vi "ShoreDefinition3.vi"(0 "Image In":T1, 7 "error in":errorcluster) -> (20 "Image Out":T1, 27 "error out":errorcluster)   [LabVIEW 2014]
uses:
  <vilib>/vision/Image Controls.llb/IMAQ Image.ctl
  <vilib>/vision/NI_Vision_Development_Module.lvlib
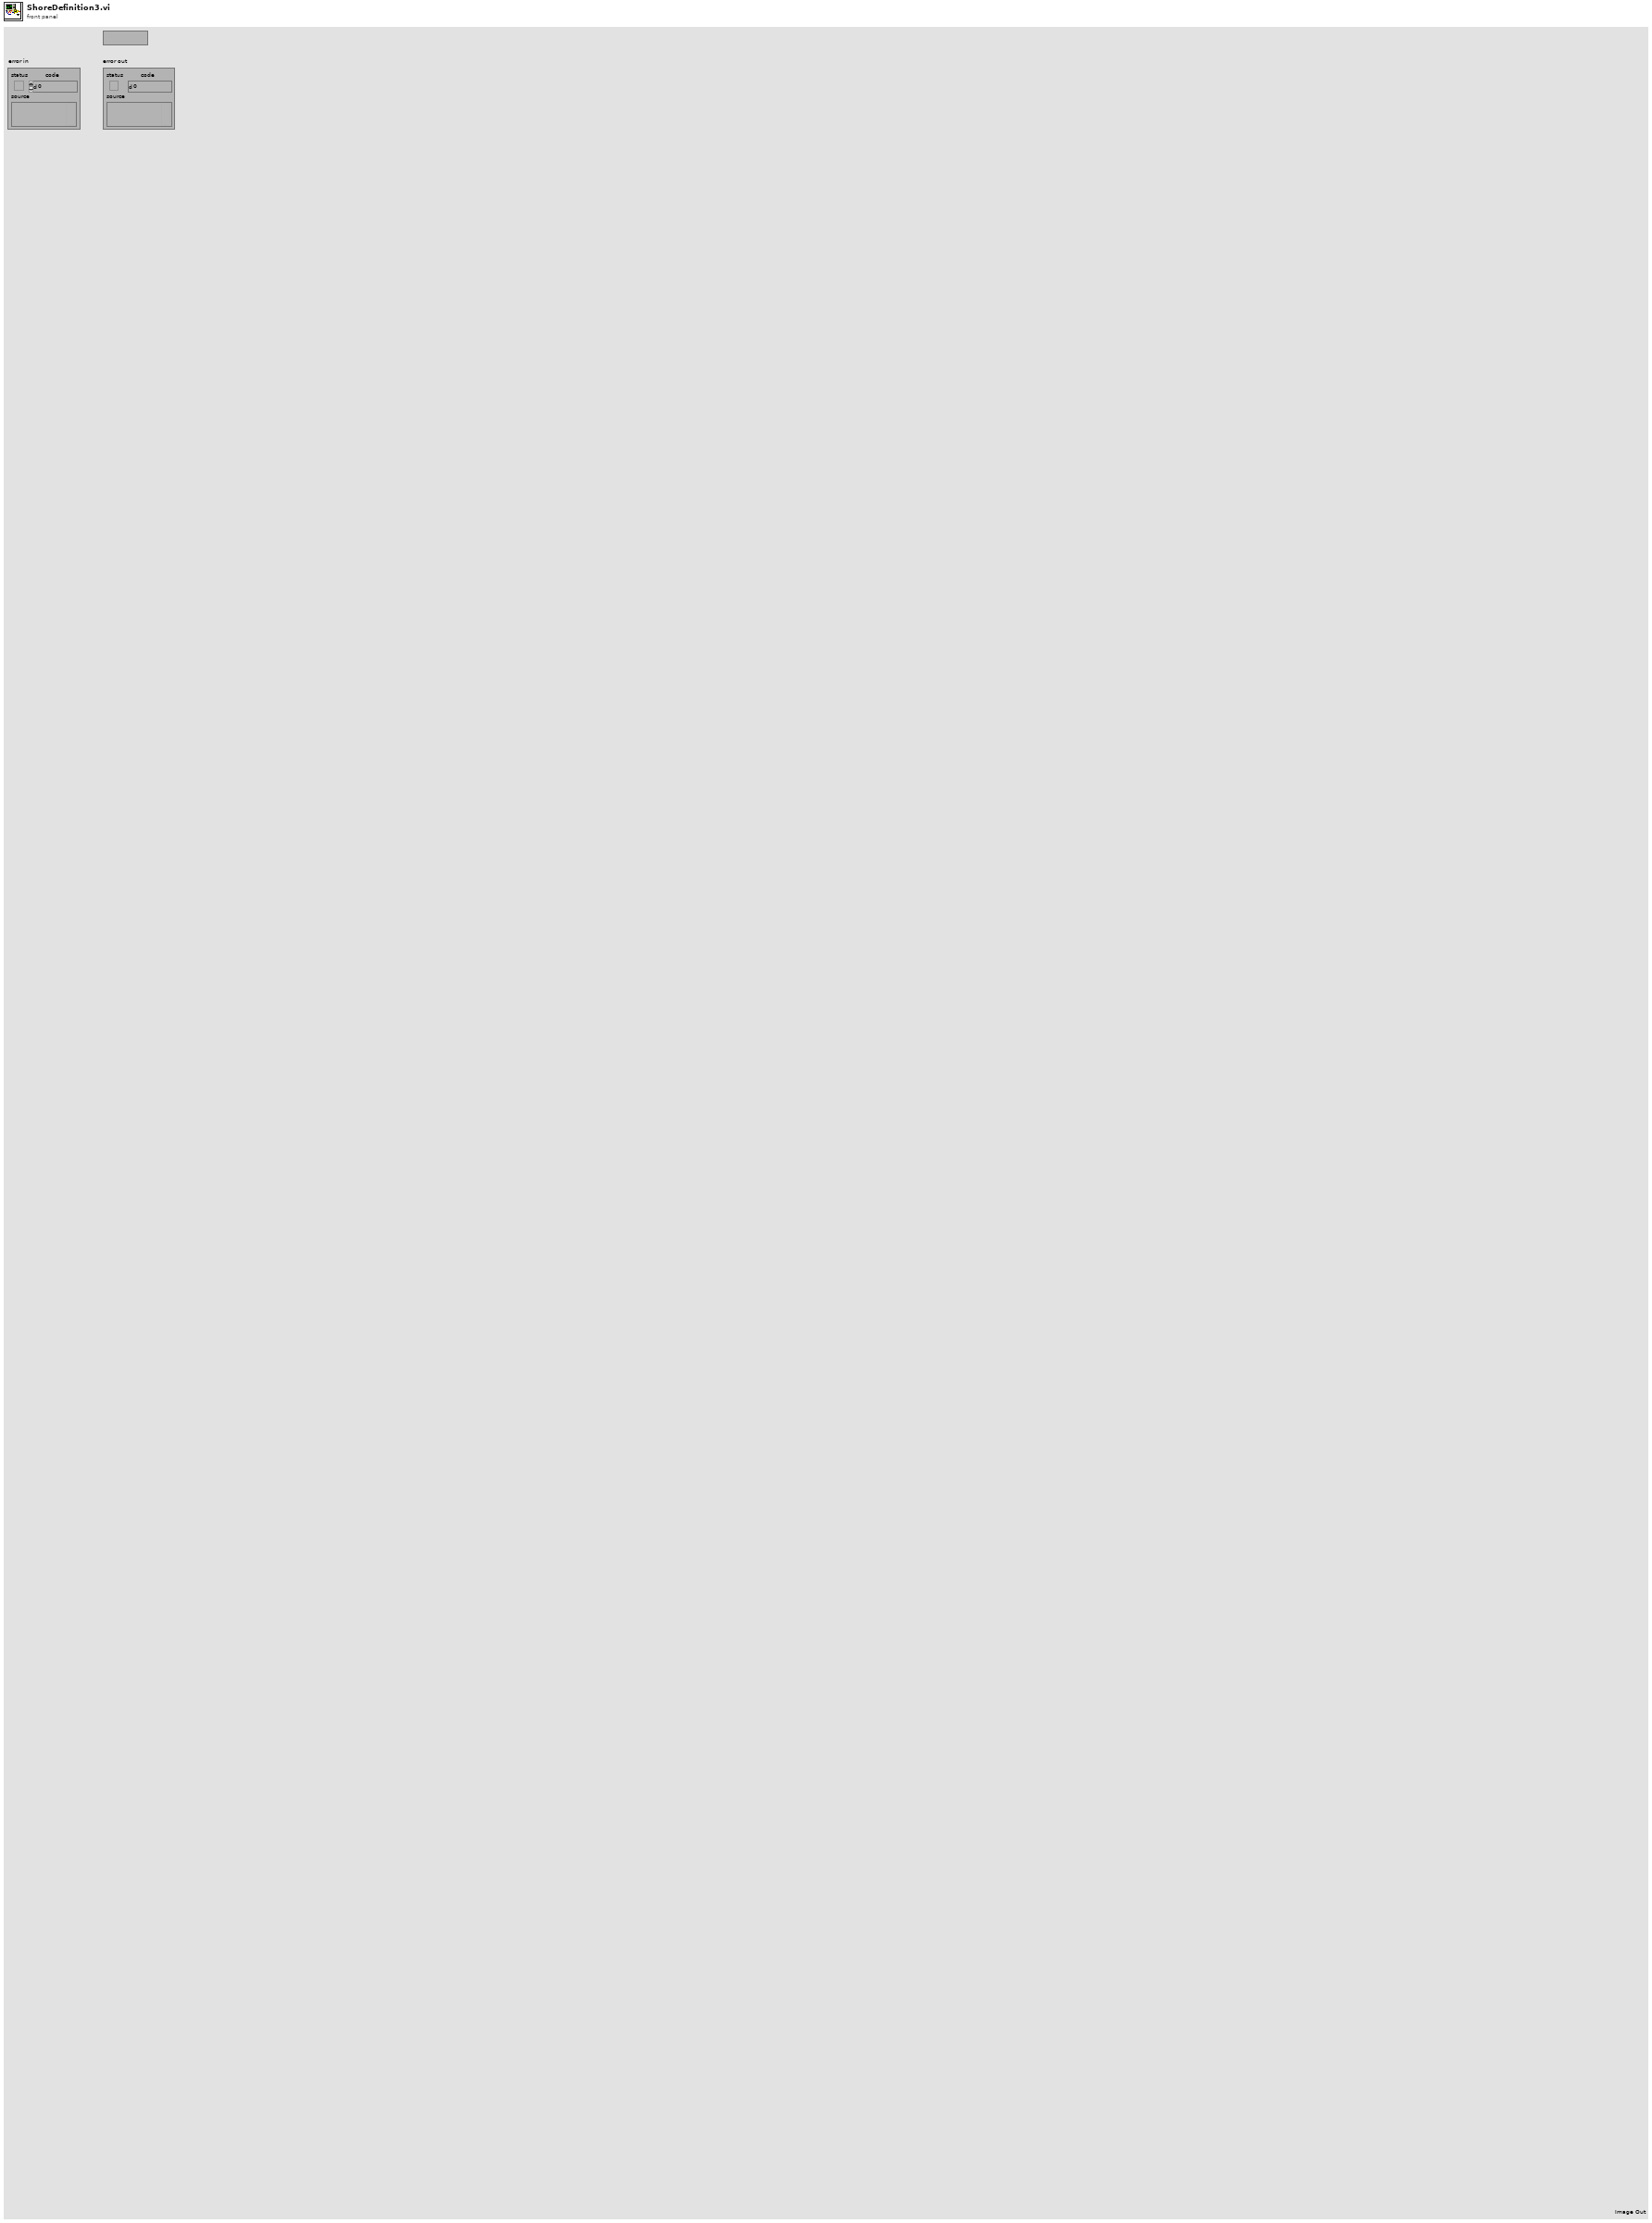
[diagram p1: front panel]
types:
  T1 = typedef "IMAQ Image.ctl" = refnum<image>
  T2 = enum32{"AutoM", "Close", "Dilate", "Erode", "Gradient", "Gradient out", "Gradient in", "Hit miss", "Open", "PClose", "POpen", "Thick", "Thin"}
  T3 = typedef "Image Type" = u32
  T4 = cluster{"Brightness":sgl, "Contrast":sgl, "Gamma":sgl}
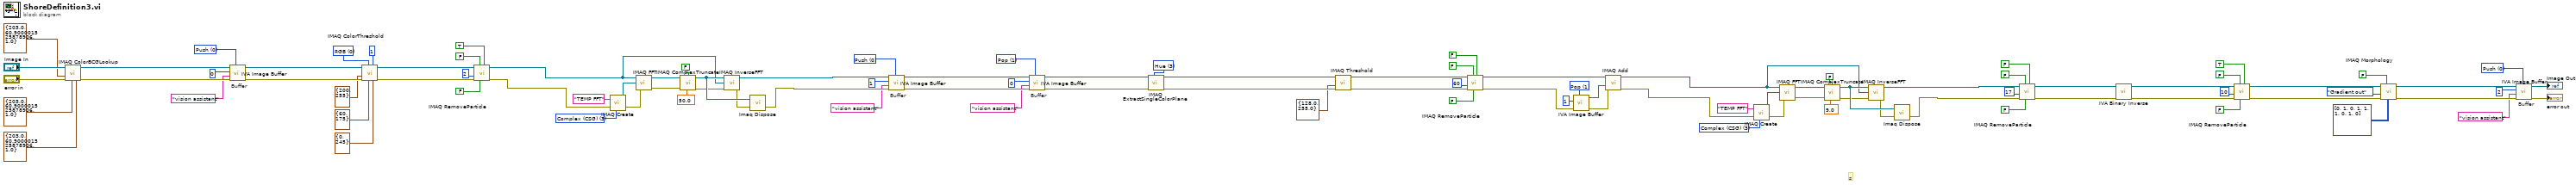
[diagram p0: block diagram]
diagram:
  w4 = u16 0 items=["Push", "Pop", "Reset"] ("Function")
  w26 = T3 3 items=["Grayscale (U8)", "Grayscale (I16)", "Grayscale (SGL)", "Complex (CSG)", "RGB (U32)", "HSL (U32)", "RGB (U64)", "Grayscale (U16)"] ("Image Type")
  w44 = u16 1 items=["Push", "Pop", "Reset"] ("Function")
  w56 = 3 items=["Red", "Green", "Blue", "Hue", "Saturation", "Luminance", "Value", "Intensity"] ("Color Plane")
  w59 = u16 1 items=["Push", "Pop", "Reset"] ("Function")
  w64 = u16 0 items=["Push", "Pop", "Reset"] ("Function")
  w67 = T3 3 items=["Grayscale (U8)", "Grayscale (I16)", "Grayscale (SGL)", "Complex (CSG)", "RGB (U32)", "HSL (U32)", "RGB (U64)", "Grayscale (U16)"] ("Image Type")
  w91 = u16 0 items=["RGB", "HSL", "HSV", "HSI"] ("Color Mode")
  w95 = u16 0 items=["Push", "Pop", "Reset"] ("Function")
  # "s"
  # "Buffer"
  # "Buffer"
  # "Buffer"
  # "Buffer"
  n1 = call "IMAQ ColorBCGLookup"("Blue BCG Values"=T4 {"Brightness"=203.0, "Contrast"=60.9, "Gamma"=1.0}, "Green BCG Values"=T4 {"Brightness"=203.0, "Contrast"=60.9, "Gamma"=1.0}, "error in (no error)"="error in", "Red BCG Values"=T4 {"Brightness"=203.0, "Contrast"=60.9, "Gamma"=1.0}, "Image Src"="Image In") -> ("error out"=w101:errorcluster, "Image Dst Out"=w97:T1)  [unwired: 2 in, 3 out]
  n2 = call <vilib>:"IVA Image Buffer.vi"("Function"=w95, "error in (no error)"=w101, "Prefix"="vision assistant", "Buffer #"=0, "Image In"=w97) -> ("error out"=w96:errorcluster, "Image Out"=w87:T1)  [unwired: 5 out]
  n3 = call "IMAQ ColorThreshold"("Blue or Luma or Val or Inten Range"=cluster{"Lower value":i32, "Upper value":i32} {"Lower value"=0, "Upper value"=245}, "Replace Value"=1, "Green or Sat Range"=cluster{"Lower value":i32, "Upper value":i32} {"Lower value"=60, "Upper value"=175}, "Color Mode"=w91, "error in (no error)"=w96, "Red or Hue Range"=cluster{"Lower value":i32, "Upper value":i32} {"Lower value"=200, "Upper value"=255}, "Image Src"=w87) -> ("error out"=w86:errorcluster, "Image Dst Out"=w81:T1)  [unwired: 1 in, 2 out]
  n4 = call "IMAQ RemoveParticle"("Connectivity 4/8 (8)"=TRUE, "Low Pass/High Pass (Low)"=FALSE, "Square/Hexa (Square)"=FALSE, "error in (no error)"=w86, "Number of Erosion"=2, "Image Src"=w81) -> ("error out"=w80:errorcluster, "Image Dst Out"=w70:T1)  [unwired: 1 in, 3 out]
  n5 = call "IMAQ Create"("Image Name"="TEMP FFT", "Image Type"=w67, "error in (no error)"=w80) -> ("New Image"=w78:T1, "error out"=w71:errorcluster)  [unwired: 1 in, 1 out]
  n6 = call "IMAQ FFT"("error in (no error)"=w71, "Image Dst"=w78, "Image Src"=w70) -> ("error out"=w76:errorcluster, "Image Dst Out"=w77:T1)  [unwired: 1 out]
  n7 = call "IMAQ ComplexTruncate"("error in (no error)"=w76, "Truncation Frequency %"=sgl 50.0, "Image Src"=w77, "Low pass/High pass (Low pass)"=FALSE) -> ("error out"=w74:errorcluster, "Image Dst Out"=w75:T1)  [unwired: 1 in, 2 out]
  n8 = call "IMAQ InverseFFT"("error in (no error)"=w74, "Image Dst"=w70, "Image Src"=w75) -> ("error out"=w73:errorcluster, "Image Dst Out"=w66:T1)  [unwired: 1 out]
  n9 = call "Imaq Dispose"("Image"=w75, "error in (no error)"=w73) -> ("error out"=w72:errorcluster)  [unwired: 1 in, 3 out]
  n10 = call <vilib>:"IVA Image Buffer.vi"("Function"=w64, "error in (no error)"=w72, "Prefix"="vision assistant", "Buffer #"=1, "Image In"=w66) -> ("error out"=w65:errorcluster, "Image Out"=w61:T1)  [unwired: 5 out]
  n11 = call <vilib>:"IVA Image Buffer.vi"("Function"=w59, "error in (no error)"=w65, "Prefix"="vision assistant", "Buffer #"=0, "Image In"=w61) -> ("error out"=w60:errorcluster, "Image Out"=w55:T1)  [unwired: 5 out]
  n12 = call "IMAQ ExtractSingleColorPlane"("Color Plane"=w56, "error in (no error)"=w60, "Image Src"=w55) -> ("error out"=w54:errorcluster, "Image Dst Out"=w52:T1)  [unwired: 1 in, 6 out]
  n13 = call "IMAQ Threshold"("error in (no error)"=w54, "Range"=cluster{"Lower value":sgl, "Upper value":sgl} {"Lower value"=128.0, "Upper value"=255.0}, "Image Src"=w52) -> ("error out"=w51:errorcluster, "Image Dst Out"=w46:T1)  [unwired: 3 in, 4 out]
  n14 = call "IMAQ RemoveParticle"("Connectivity 4/8 (8)"=FALSE, "Low Pass/High Pass (Low)"=FALSE, "Square/Hexa (Square)"=FALSE, "error in (no error)"=w51, "Number of Erosion"=60, "Image Src"=w46) -> ("error out"=w45:errorcluster, "Image Dst Out"=w41:T1)  [unwired: 1 in, 3 out]
  n15 = call <vilib>:"IVA Image Buffer.vi"("Function"=w44, "error in (no error)"=w45, "Buffer #"=1) -> ("error out"=w40:errorcluster, "Image Out"=w42:T1)  [unwired: 2 in, 5 out]
  n16 = call "IMAQ Add"("Image Src A"=w41, "Image Src B"=w42, "error in (no error)"=w40) -> ("Image Dst Out"=w29:T1, "error out"=w39:errorcluster)  [unwired: 2 in, 2 out]
  n17 = call "IMAQ Create"("Image Name"="TEMP FFT", "Image Type"=w26, "error in (no error)"=w39) -> ("New Image"=w37:T1, "error out"=w30:errorcluster)  [unwired: 1 in, 1 out]
  n18 = call "IMAQ FFT"("error in (no error)"=w30, "Image Dst"=w37, "Image Src"=w29) -> ("error out"=w35:errorcluster, "Image Dst Out"=w36:T1)  [unwired: 1 out]
  n19 = call "IMAQ ComplexTruncate"("error in (no error)"=w35, "Truncation Frequency %"=sgl 9.0, "Image Src"=w36, "Low pass/High pass (Low pass)"=FALSE) -> ("error out"=w33:errorcluster, "Image Dst Out"=w34:T1)  [unwired: 1 in, 2 out]
  n20 = call "IMAQ InverseFFT"("error in (no error)"=w33, "Image Dst"=w29, "Image Src"=w34) -> ("error out"=w32:errorcluster, "Image Dst Out"=w21:T1)  [unwired: 1 out]
  n21 = call "Imaq Dispose"("Image"=w34, "error in (no error)"=w32) -> ("error out"=w31:errorcluster)  [unwired: 1 in, 3 out]
  n22 = call "IMAQ RemoveParticle"("Connectivity 4/8 (8)"=FALSE, "Low Pass/High Pass (Low)"=FALSE, "Square/Hexa (Square)"=FALSE, "error in (no error)"=w31, "Number of Erosion"=17, "Image Src"=w21) -> ("error out"=w20:errorcluster, "Image Dst Out"=w19:T1)  [unwired: 1 in, 3 out]
  n23 = call <vilib>:"IVA Binary Inverse.vi"("error in (no error)"=w20, "Image In"=w19) -> ("error out"=w18:errorcluster, "Image Out"=w13:T1)  [unwired: 8 out]
  n24 = call "IMAQ RemoveParticle"("Connectivity 4/8 (8)"=TRUE, "Low Pass/High Pass (Low)"=FALSE, "Square/Hexa (Square)"=FALSE, "error in (no error)"=w18, "Number of Erosion"=10, "Image Src"=w13) -> ("error out"=w12:errorcluster, "Image Dst Out"=w8:T1)  [unwired: 1 in, 3 out]
  n25 = call "IMAQ Morphology"("Structuring Element"=i32[][] [[0, 1, 0], [1, 1, 1], [0, 1, 0]], "Square/Hexa (Square)"=FALSE, "error in (no error)"=w12, "Operation"=T2."Gradient out", "Image Src"=w8) -> ("error out"=w7:errorcluster, "Image Dst Out"=w6:T1)  [unwired: 2 in, 3 out]
  n26 = call <vilib>:"IVA Image Buffer.vi"("Function"=w4, "error in (no error)"=w7, "Prefix"="vision assistant", "Buffer #"=2, "Image In"=w6) -> ("error out"=→"error out":errorcluster, "Image Out"=→"Image Out":T1)  [unwired: 5 out]
